vi "CMD.vi"(8 "error in (no error)":errorcluster, 10 "Command":string) -> (0 "error out":errorcluster)   [LabVIEW 2018, in "MQTT Messages.lvlib"]
uses:
  MQTT Messages.lvlib
  MQTT_Singleton/MQTT_Singleton.lvlib
panel:
  out "JSON string":string
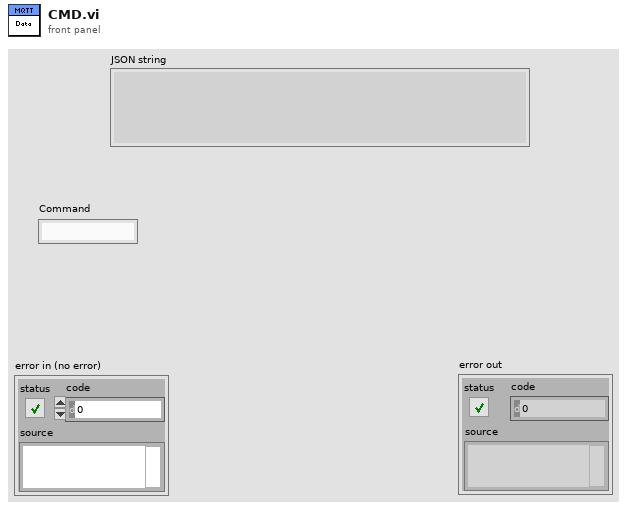
[diagram p1: front panel]
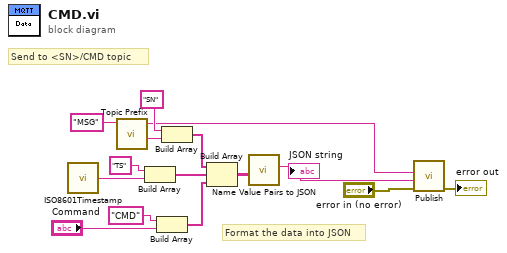
[diagram p0: block diagram]
diagram:
  # "Format the data into JSON"
  # "Send to <SN>/CMD topic"
  n1 = call "ISO8601Timestamp.vi"() -> ("date/time string"=w6:string)  [unwired: 5 in]
  n2 = call "Topic Prefix.vi"("Topic"="MSG" ("string")) -> ("SN"=w4:string, "Topic"=w2:string)  [unwired: 9 in]
  n3 = Build Array("TS" ("element"), w6) -> (w11:string[])
  n4 = Build Array("CMD" ("element"), "Command") -> (w12:string[])
  n5 = Build Array("SN" ("element"), w4) -> (w10:string[])
  n6 = Build Array(w10, w11, w12) -> (w13:string[][])
  n7 = call "Name Value Pairs to JSON.vi"("Message"=w13) -> ("JSON string"=w1:string)  [unwired: 10 in]
  "JSON string" <- w1
  n8 = call "Publish.vi"("error in (no error)"="error in (no error)", "Message"=w1, "Topic"=w2) -> ("error out"=→"error out":errorcluster)  [unwired: 8 in]
